vi "BESSY Put Test Scalar.vi"() -> ()   [LabVIEW 2011]
doc: "This Arbitrary Waveform Generator front panel is aimed primarily at the use of two reflectometer instruments at the ISIS Pulsed Neutron Facility at the Rutherford Appleton Laboratory. As such some variable items have been defaulted, and the code follows the standards of the Instrument Controls programming team."
uses:
  Labview Modules/Common/Utilities/Logo.llb/Logo.ctl
  Labview Modules/Common/Utilities/VI Control.llb/Control - Display State.ctl
  Labview Modules/Drivers/Tektronix AFG 3021B/AFG3021B - Controls.llb/AFG3021B - Trigger Button.ctl
  <userlib>/caLab/sub/caLabGet02.vi
  Labview Modules/Common/Utilities/Equal.llb/Equal - Error.vi
  <userlib>/caLab/sub/caLabPut41.vi
panel:
  out "Set Point Ind":dbl
  in  "Set Point":dbl
  in  "Exit":bool
  in  "Set":bool
  out "Message":string
  out "Activity":bool
  out "Error":errorcluster
  in  "Logo":T1
  # "Version 0.0.1"
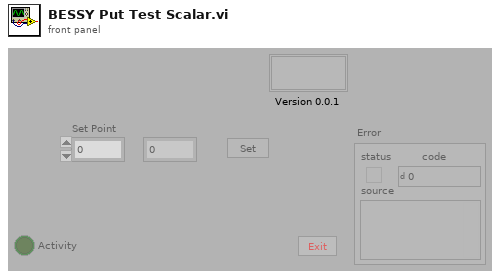
[diagram p1: front panel]
types:
  T1 = typedef "Logo.ctl" = u16
  T2 = typedef "Control - Display State.ctl" = enum16{"Enabled", "Disabled", "Disabled and Grayed"}
  T3 = typedef "AFG3021B - Trigger Button.ctl" = bool
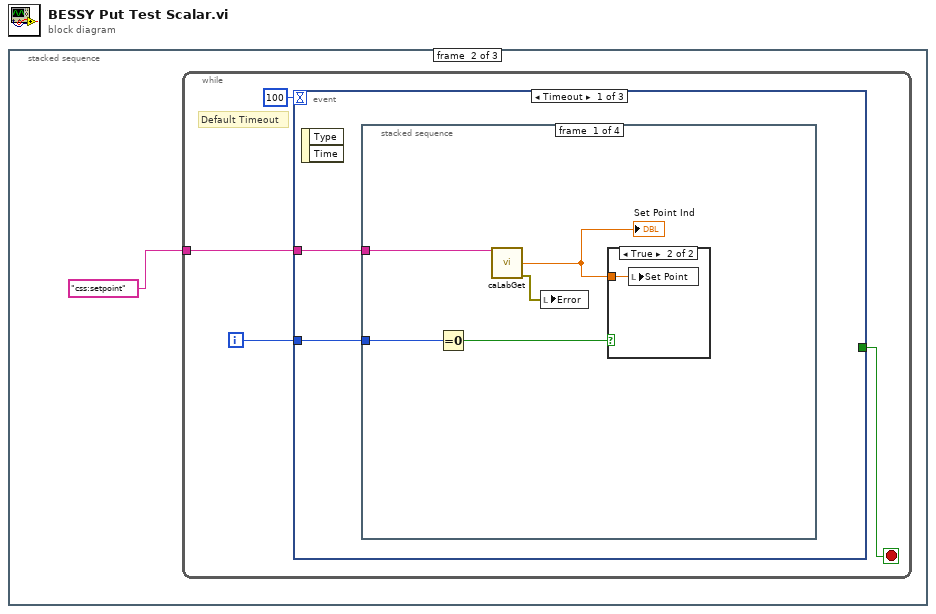
[diagram p0: block diagram]
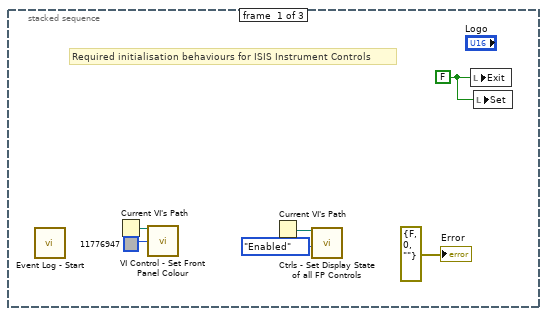
[diagram p2: hidden frame]
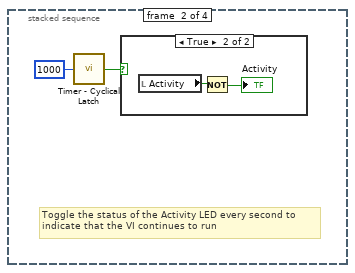
[diagram p4: hidden frame]
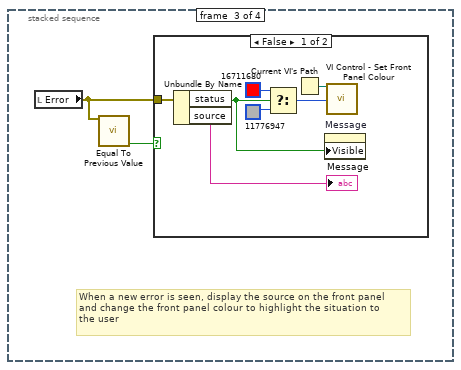
[diagram p6: hidden frame]
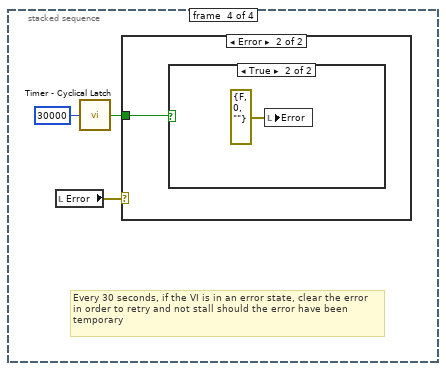
[diagram p8: hidden frame]
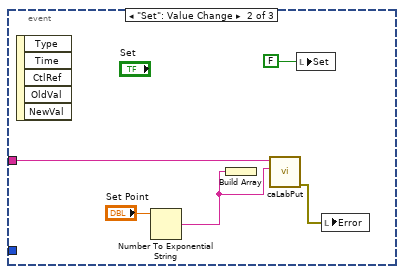
[diagram p11: hidden frame]
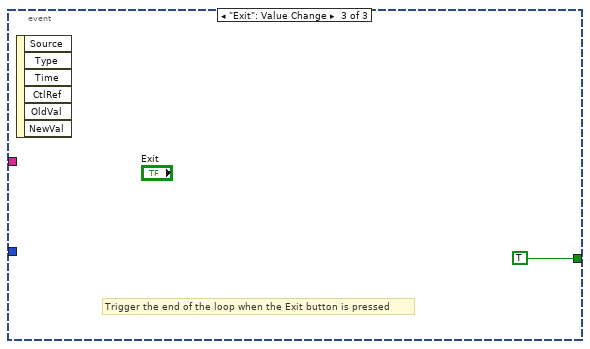
[diagram p12: hidden frame]
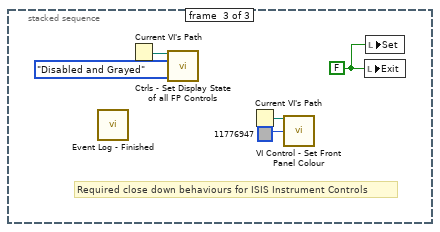
[diagram p13: hidden frame]
diagram:
  n1 = stacked-sequence {
    frame #0 {
      w1 = FALSE
      # "Required initialisation behaviours for ISIS Instrument Controls"
      n2 = call "Event Log - Start.vi"() -> ()  [unwired: 1 in]
      n3 = Current VI's Path() -> (path=w2:path)
      n4 = call "VI Control - Set Front Panel Colour.vi"("VI Path"=w2, "Front Panel Colour"=u32 11776947) -> ()  [unwired: 13 in, 1 out]
      n5 = Current VI's Path() -> (path=w6:path)
      n6 = call "Ctrls - Set Display State of all FP Controls.vi"("VI Path"=w6, "Display State"=Control_-_Display_State."Enabled") -> ()  [unwired: 18 in]
      n7 = local write "Exit"(w1) -> ()
      n8 = local write "Set"(w1) -> ()
      "Error" <- errorcluster {"status"=FALSE, "code"=0, "source"=""} ("Error")
    }
    frame #1 {
      n9 = while {
        tunnel: "css:setpoint" ("PV name") -> [w8]
        i -> [w9]
        stop <- w10 stop-if-true
        # "Default Timeout"
        n10 = event shown="[0] Timeout" {
          selector: _ -> [_ _ _]
          dyn-events: _ -> [_ _ _]
          timeout: 100 -> [_ _ _]
          tunnel: [_ _ TRUE] -> w10
          tunnel: w9 -> [w13 _ _]
          tunnel: w8 -> [w12 w41 _]
          event Timeout {
            n11 = event-data() -> ()  [unwired: 1 in, 2 out]
            n12 = stacked-sequence {
              tunnel: w13 -> [w18 _ _ _]
              tunnel: w12 -> [w15 _ _ _]
              frame #0 {
                n13 = Equal To 0?(x=w18) -> (x = 0?=w17:bool)
                n14 = call-poly <userlib>:"caLabGet.vi"("PV name"=w15) -> ("1st value(number)"=w14:dbl, "error out"=w16:errorcluster)  [unwired: 8 in, 5 out]
                "Set Point Ind" <- w14
                n15 = local write "Error"(w16) -> ()
                n16 = case shown="True" w17 {
                  tunnel: w14 -> [_ w19]
                  frame False {
                  }
                  frame True {
                    n17 = local write "Set Point"(w19) -> ()
                  }
                }
              }
              frame #1 {
                # "Toggle the status of the Activity LED every second to\nindicate that the VI continues to run"
                n18 = call "Timer - Cyclical Latch.vi"("Timer (msec)"=u32 1000) -> ("Timer Trigger"=w20:bool)  [unwired: 14 in]
                n19 = case shown="True" w20 {
                  frame False {
                  }
                  frame True {
                    n20 = local read "Activity"() -> (w22:bool)
                    n21 = Not(x=w22) -> (.not. x?=→"Activity":bool)
                  }
                }
              }
              frame #2 {
                # "When a new error is seen, display the source on the front panel\nand change the front panel colour to highlight the situation to\nthe user"
                n22 = local read "Error"() -> (w25:errorcluster)
                n23 = call-poly "Equal To Previous Value.vi"("Value In"=w25) -> ("Equal to previous value"=w24:bool)  [unwired: 13 in, 1 out]
                n24 = case shown="False" w24 {
                  tunnel: w25 -> [w28 _]
                  frame False {
                    n25 = Unbundle By Name(w28) -> ("status"=w27:bool, "source"=→"Message":string)
                    n26 = Select(t=u32 16711680, s=w27, f=u32 11776947) -> (s? t:f=w29:u32)
                    n27 = Current VI's Path() -> (path=w32:path)
                    n28 = property on="Message" class="Str"("Visible"=w27) -> ()  [unwired: 2 in, 2 out]
                    n29 = call "VI Control - Set Front Panel Colour.vi"("VI Path"=w32, "Front Panel Colour"=w29) -> ()  [unwired: 13 in, 1 out]
                  }
                  frame True {
                  }
                }
              }
              frame #3 {
                # "Every 30 seconds, if the VI is in an error state, clear the error\nin order to retry and not stall should the error have been \ntemporary"
                n30 = local read "Error"() -> (w34:errorcluster)
                n31 = call "Timer - Cyclical Latch.vi"("Timer (msec)"=u32 30000) -> ("Timer Trigger"=w33:bool)  [unwired: 14 in]
                n32 = case shown="Error" w34 {
                  tunnel: w33 -> [_ w36]
                  frame No Error {
                  }
                  frame Error {
                    n33 = case shown="True" w36 {
                      frame False {
                      }
                      frame True {
                        n34 = local write "Error"(errorcluster {"status"=FALSE, "code"=0, "source"=""} ("Error")) -> ()
                      }
                    }
                  }
                }
              }
            }
          }
          event "Set": Value Change {
            n35 = event-data() -> ()  [unwired: 1 in, 5 out]
            n36 = Number To Exponential String(number="Set Point") -> (E-format string=w38:string)  [unwired: 3 in]
            n37 = Build Array(w38) -> ()  [unwired: 1 out]
            n38 = call-poly <userlib>:"caLabPut.vi"("values"=w38, "PV name(s)"=w41) -> ("error out"=w40:errorcluster)  [unwired: 6 in, 3 out]
            n39 = local write "Set"(T3 FALSE ("Trigger")) -> ()
            n40 = local write "Error"(w40) -> ()
          }
          event "Exit": Value Change {
            # "Trigger the end of the loop when the Exit button is pressed"
            n41 = event-data() -> ()  [unwired: 1 in, 6 out]
          }
        }
      }
    }
    frame #2 {
      w44 = FALSE
      # "Required close down behaviours for ISIS Instrument Controls"
      n42 = call "Event Log - Finished.vi"() -> ()  [unwired: 1 in]
      n43 = Current VI's Path() -> (path=w47:path)
      n44 = call "Ctrls - Set Display State of all FP Controls.vi"("VI Path"=w47, "Display State"=Control_-_Display_State."Disabled and Grayed") -> ()  [unwired: 18 in]
      n45 = Current VI's Path() -> (path=w46:path)
      n46 = call "VI Control - Set Front Panel Colour.vi"("VI Path"=w46, "Front Panel Colour"=u32 11776947) -> ()  [unwired: 13 in, 1 out]
      n47 = local write "Exit"(w44) -> ()
      n48 = local write "Set"(w44) -> ()
    }
  }
